vi "Read Boolean.vi"(8 "error in (no error)":errorcluster, 11 "Event in":refnum<class "Event Boolean.lvclass">) -> (0 "error out":errorcluster, 2 "Boolean":bool, 3 "Event out":refnum<class "Event Boolean.lvclass">)   [LabVIEW 2017, in "Event Actors.lvlib" / "Event Boolean.lvclass"]
uses:
  Event Boolean.lvclass
  Event Boolean.lvclass/Event Boolean.ctl
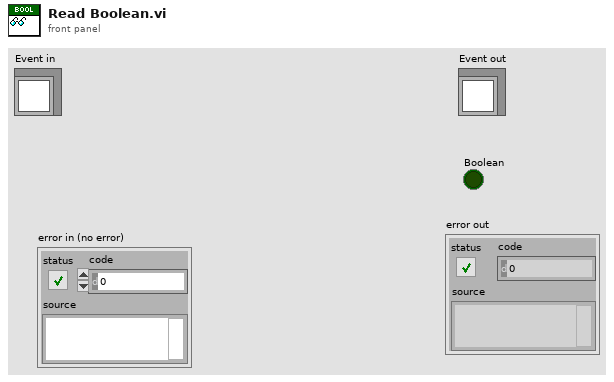
[diagram p1: front panel]
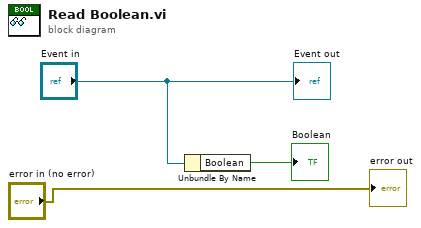
[diagram p0: block diagram]
diagram:
  n1 = Unbundle By Name("Event in") -> ("Boolean"=→"Boolean":bool)
  "Event out" <- "Event in"
  "error out" <- "error in (no error)"
